vi "Suggest New Attribute ID.vi"() -> ()   [LabVIEW 2023]
uses:
  <vilib>/Utility/file.llb/Read Delimited Spreadsheet (string).vi
panel:
  out "Waveform Graph":u32[](graph)
  out "error out":errorcluster
  out "Number of IDs found":i32
  out "Last ID used":string
  out "Suggested New ID":string
  in  "file path":path=path "E:/Dev/ni-central/src/rfmx/SpecAn/RFmxSpecAnLV/source/resource/objmgr/RFmxSpecAnAttributes.xml"
  # "Select the attributes xml file path and run the program"
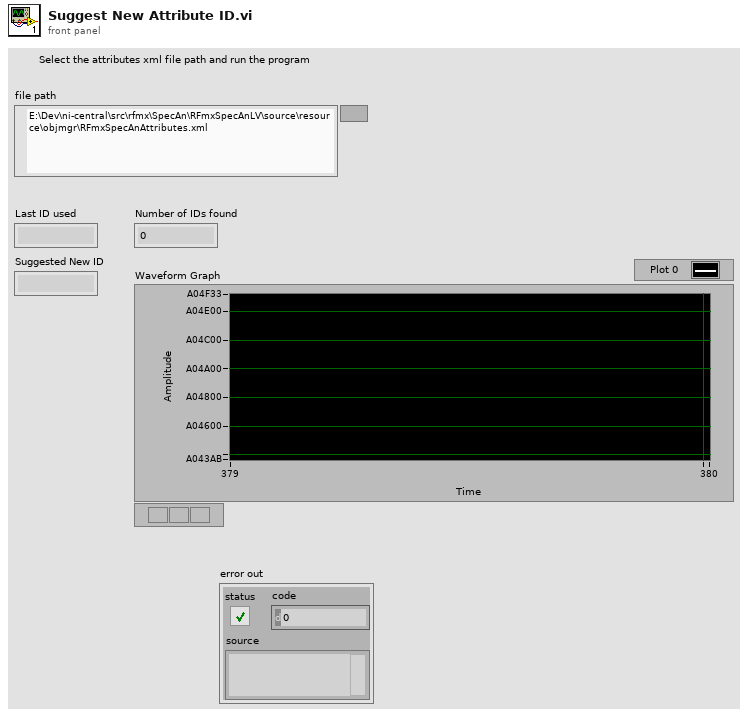
[diagram p1: front panel]
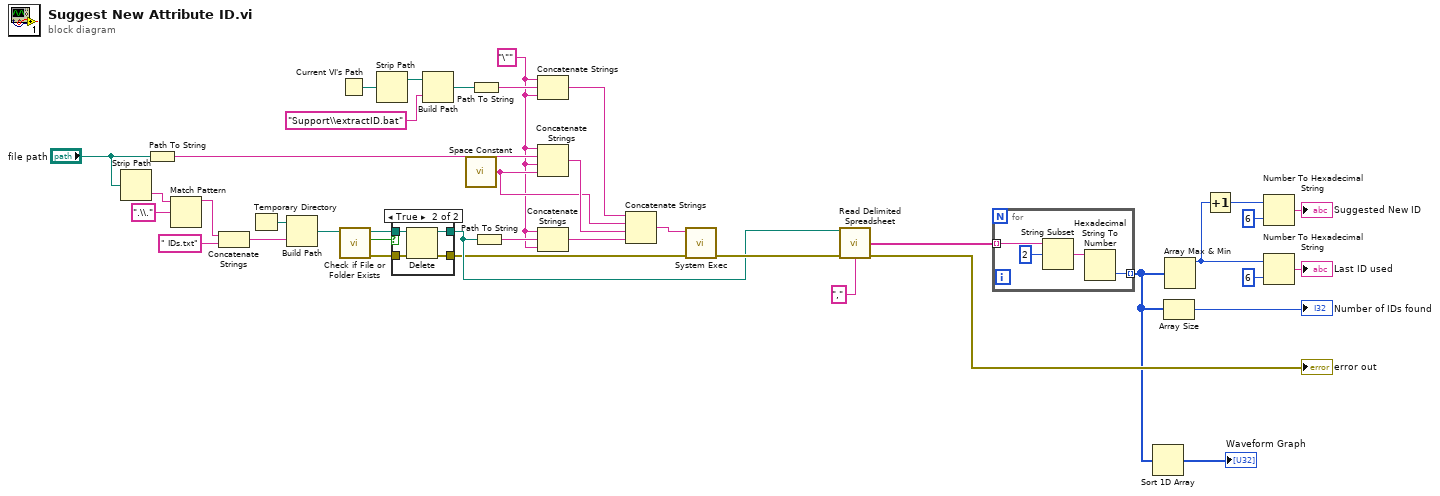
[diagram p0: block diagram]
diagram:
  w6 = "\"" ("string")
  n1 = Strip Path(path="file path") -> (name=w16:string)  [unwired: 1 out]
  n2 = Path To String(path="file path") -> (string=w39:string)
  n3 = Match Pattern(string=w16, regular expression=".\\.") -> (before substring=w15:string)  [unwired: 1 in, 3 out]
  n4 = Concatenate Strings(w15, " IDs.txt" ("string")) -> (w14:string)
  n5 = Temporary Directory() -> (w38:path)
  n6 = Build Path(base path=w38, name or relative path=w14) -> (appended path=w23:path)
  n7 = Current VI's Path() -> (path=w12:path)
  n8 = call <vilib>:"Check if File or Folder Exists.vi"("path"=w23) -> ("error out"=w20:errorcluster, "file or folder exists?"=w21:bool, "dup path"=w22:path)  [unwired: 8 in]
  n9 = Strip Path(path=w12) -> (stripped path=w10:path)  [unwired: 1 out]
  n10 = case shown="True" w21 {
    tunnel: w22 -> [w41 w45]
    tunnel: [w41 w44] -> w13
    tunnel: w20 -> [w40 w43]
    tunnel: [w40 w42] -> w5
    frame False {
    }
    frame True {
      n11 = Delete(path (use dialog)=w45, error in=w43) -> (deleted path=w44:path, error out=w42:errorcluster)  [unwired: 3 in, 1 out]
    }
  }
  n12 = Build Path(base path=w10, name or relative path="Support\\extractID.bat" ("string")) -> (appended path=w9:path)
  n13 = call <vilib>:"Space Constant.vi"() -> ("String"=w33:string)
  n14 = Path To String(path=w9) -> (string=w8:string)
  n15 = Path To String(path=w13) -> (string=w37:string)
  n16 = Concatenate Strings(w6, w8, w6) -> (w7:string)
  n17 = Concatenate Strings(w6, w39, w6, w33) -> (w35:string)
  n18 = Concatenate Strings(w6, w37, w6) -> (w36:string)
  n19 = Concatenate Strings(w7, w33, w35, w36) -> (w34:string)
  n20 = call <vilib>:"System Exec.vi"("error in (no error)"=w5, "command line"=w34) -> ("error out"=w24:errorcluster)  [unwired: 6 in, 3 out]
  n21 = call-poly <vilib>:"Read Delimited Spreadsheet.vi"("file path (dialog if empty)"=w13, "error in (no error)"=w24, "delimiter (\\t)"="," ("delimiter (\\t)")) -> ("first row"=w4:string[], "error out"=→"error out":errorcluster)  [unwired: 7 in, 4 out]
  n22 = for {
    tunnel: w4 -> [w49] mode=indexing
    tunnel: [w47] -> w2 mode=indexing
    n23 = String Subset(string=w49, offset (0)=2) -> (substring=w46:string)  [unwired: 1 in]
    n24 = Hexadecimal String To Number(string=w46) -> (number=w47:u32)  [unwired: 2 in, 1 out]
  }
  n25 = Sort 1D Array(array=w2) -> (sorted array=→"Waveform Graph":u32[])
  n26 = Array Size(array=w2) -> (size(s)=→"Number of IDs found":i32)
  n27 = Array Max & Min(array=w2) -> (max value=w26:u32)  [unwired: 3 out]
  n28 = Increment(x=w26) -> (x+1=w31:u32)
  n29 = Number To Hexadecimal String(1:i16 6 ("width (-)"), 2:w31) -> (0:→"Suggested New ID":string)
  n30 = Number To Hexadecimal String(1:i16 6 ("width (-)"), 2:w26) -> (0:→"Last ID used":string)
